vi "cblas zdotc.vi"(5 "n":i32=-1, 6 "incy":i32=1, 7 "incx":i32=1, 10 "y":cdb[](array[numeric]), 11 "x":cdb[](array[numeric])) -> (0 "error":i32, 3 "zdotc":cdb)   [LabVIEW 2018, in "NI_AALBLAS.lvlib"]
uses:
  NI_AALBLAS.lvlib
  Operation_Conjugate.ctl
  <resource>/lvblas.dll
panel:
  # "void cblas_zdotc_sub(n, *x, incx, *y, incy, *zdotc)"
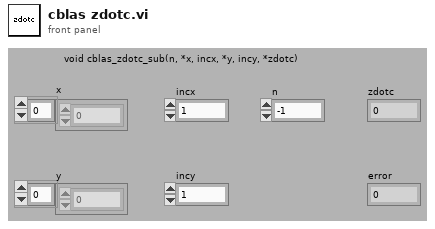
[diagram p1: front panel]
types:
  T1 = typedef "NI_AALBLAS.lvlib/Operation_Conjugate.ctl" = i32
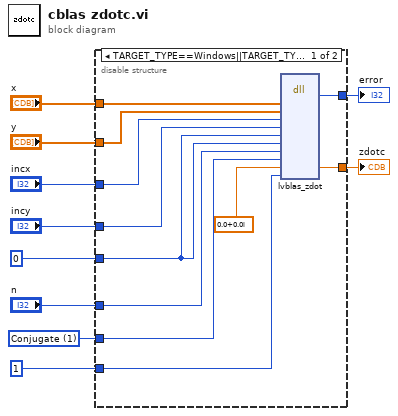
[diagram p0: block diagram]
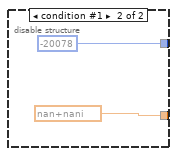
[diagram p2: hidden frame]
diagram:
  w6 = T1 1 items=["Not Conjugate", "Conjugate"] ("operation X")
  n1 = disable-structure shown="TARGET_TYPE==Windows||TARGET_TYPE==Unix||TARGET_TYPE==Mac||TARGET_TYPE==RT" {
    disable-tunnel: [w15 cdb nan+nani] -> w10
    disable-tunnel: "x" -> [w21 _]
    disable-tunnel: "y" -> [w20 _]
    disable-tunnel: "n" -> [w19 _]
    disable-tunnel: [w18 -20078 ("error")] -> w7
    disable-tunnel: w6 -> [w17 _]
    disable-tunnel: 0 -> [w16 _]
    disable-tunnel: "incx" -> [w13 _]
    disable-tunnel: "incy" -> [w12 _]
    disable-tunnel: 1 -> [w11 _]
    frame condition #0 (active) {
      n2 = dll-call lib="C:/Program Files (x86)/National Instruments/LabVIEW 2018/resource/lvblas.*" fn="lvblas_zdot" ("CBLAS.dll:CxDotProdH")("X"=w21, "Y"=w20, "IncX"=w13, "IncY"=w12, "startX"=w16, "startY"=w16, "N"=w19, "OpX"=w17, "DotProd"=cdb 0.0+0.0i, "check"=w11) -> ("error"=w18:i32, "DotProd"=w15:cdb)  [unwired: 12 in, 2 out]
    }
    frame condition #1 {
    }
  }
  "error" <- w7
  "zdotc" <- w10
